vi "Temporales.vi"() -> ()   [LabVIEW 2013]
panel:
  in  "Escanear":bool
  out "Salir":bool
  out "Avance":dbl
  out "Estatus":string
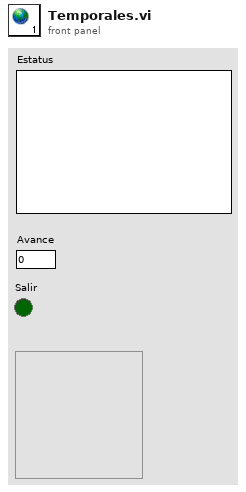
[diagram p1: front panel]
diagram:
